vi "GetXYFromTxt.vi"(8 "error in":errorcluster, 11 "path to pos.txt":path) -> (0 "error out":errorcluster, 1 "Yy":dbl, 2 "Xy":dbl, 4 "Xw":dbl, 5 "Yr":dbl, 6 "Yw":dbl, 7 "Xr":dbl)   [LabVIEW 2022 SP3]
doc: "This VI extract balls's coordinates from a text file\n\nIt first opens pos.txt that contains three lines with text, x-position, y-position and the score of each of the red, yellow and white ball, read them and converts them into DBL and then closes the file.\nIf the score is equal to 0, meaning that we didn't find the ball, the VI return a NaN.\n\n\n--/!\\-- WARNING --/!\\-- \n\nThis VI uses a predefined text organisation :\n\nRed : Xr, Yr, ScoreRed\nYellow : Xy, Yy, ScoreYellow\nWhite : Xw, Yw, ScoreWhite\n\n--/!\\-- WARNING --/!\\-- \n\nInputs :\n- The path to pos.txt\n- Error in\n\nOutputs :\n- The balls coordinates (or NaN) (DBL)\n- Error out"
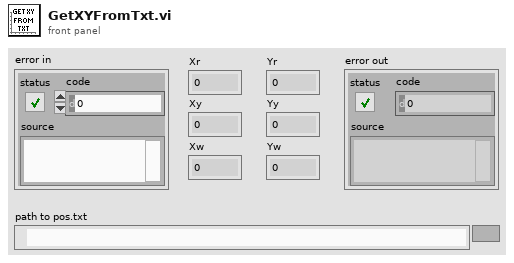
[diagram p1: front panel]
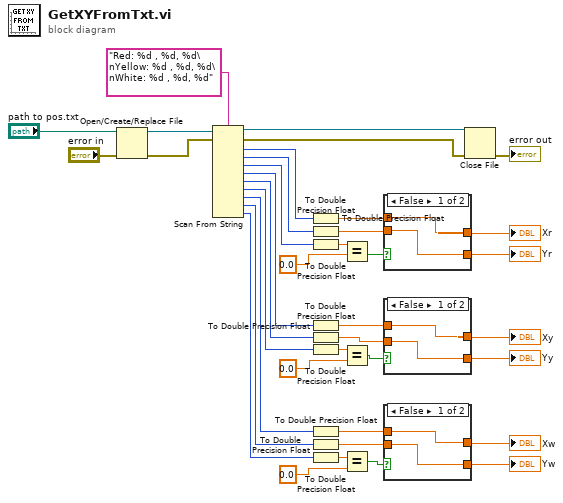
[diagram p0: block diagram]
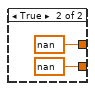
[diagram p2: hidden frame]
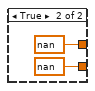
[diagram p3: hidden frame]
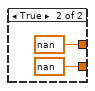
[diagram p4: hidden frame]
diagram:
  n1 = Open/Create/Replace File(file path (use dialog)="path to pos.txt", error in="error in") -> (refnum out=w23:refnum<file>, error out=w22:errorcluster)  [unwired: 4 in, 1 out]
  n2 = Scan From String ("Scan From File")("Red: %d , %d, %d\nYellow: %d , %d, %d\nWhite: %d , %d, %d" ("format string"), w23, w22) -> (w11:refnum<file>, w21:errorcluster, output 1=w20:i32, output 2=w19:i32, output 3=w18:i32, output 4=w17:i32, output 5=w16:i32, output 6=w15:i32, output 7=w14:i32, output 8=w13:i32, output 9=w12:i32)  [unwired: 9 in]
  n3 = To Double Precision Float(number=w20) -> (double precision float=w9:dbl)
  n4 = To Double Precision Float(number=w19) -> (double precision float=w8:dbl)
  n5 = To Double Precision Float(number=w18) -> (double precision float=w7:dbl)
  n6 = To Double Precision Float(number=w17) -> (double precision float=w6:dbl)
  n7 = To Double Precision Float(number=w16) -> (double precision float=w5:dbl)
  n8 = To Double Precision Float(number=w15) -> (double precision float=w4:dbl)
  n9 = To Double Precision Float(number=w14) -> (double precision float=w3:dbl)
  n10 = To Double Precision Float(number=w13) -> (double precision float=w2:dbl)
  n11 = To Double Precision Float(number=w12) -> (double precision float=w1:dbl)
  n12 = Equal?(x=w7, y=0.0) -> (x = y?=w38:bool)
  n13 = Equal?(x=w4, y=0.0) -> (x = y?=w31:bool)
  n14 = Equal?(x=w1, y=0.0) -> (x = y?=w30:bool)
  n15 = case shown="False" w38 {
    tunnel: w9 -> [w40 _]
    tunnel: w8 -> [w39 _]
    tunnel: [w40 nan] -> w36
    tunnel: [w39 nan] -> w35
    frame False {
    }
    frame True {
    }
  }
  "Xr" <- w36
  "Yr" <- w35
  n16 = case shown="False" w31 {
    tunnel: w6 -> [w44 _]
    tunnel: w5 -> [w43 _]
    tunnel: [w44 nan] -> w33
    tunnel: [w43 nan] -> w34
    frame False {
    }
    frame True {
    }
  }
  "Xy" <- w33
  "Yy" <- w34
  n17 = case shown="False" w30 {
    tunnel: w3 -> [w48 _]
    tunnel: w2 -> [w47 _]
    tunnel: [w48 nan] -> w28
    tunnel: [w47 nan] -> w27
    frame False {
    }
    frame True {
    }
  }
  "Xw" <- w28
  "Yw" <- w27
  n18 = Close File(refnum=w11, error in=w21) -> (error out=→"error out":errorcluster)  [unwired: 1 out]
